vi "open.vi"(11 "Experience ID":string="TestOK") -> (0 "error out":errorcluster, 2 "Indicators_list":T1(array[cluster]), 3 "Controls_list":T1(array[cluster]))   [LabVIEW 2014]
panel:
  out "Control Value:Get All":cluster{"Name":string, "Variant Data":variant}[](array[cluster])
  out "vi reference":refnum<vi>
  in  "OpenFP":bool=TRUE
  # "Open"
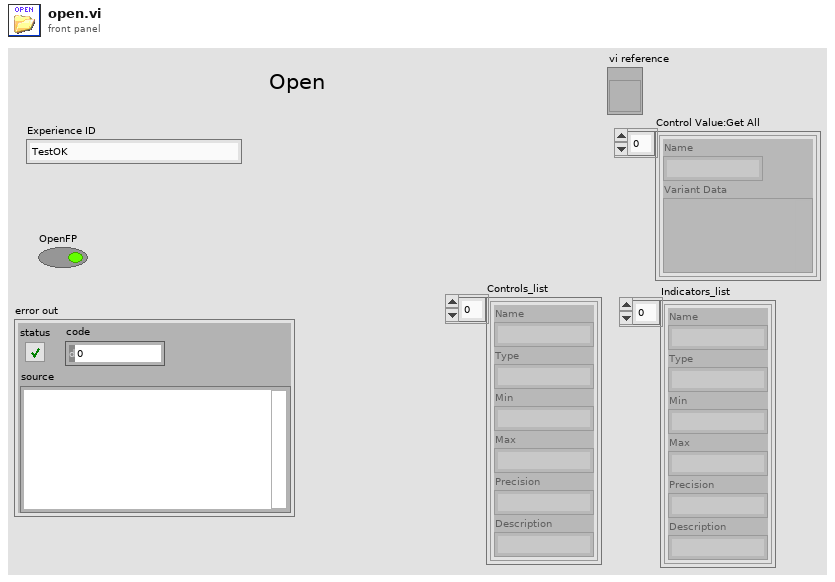
[diagram p1: front panel]
types:
  T1 = cluster{"Name":string, "Type":string, "Min":string, "Max":string, "Precision":string, "Description":string}[]
  T2 = enum32{"Invalid", "Standard", "Closed", "Hidden", "Minimized", "Maximized"}
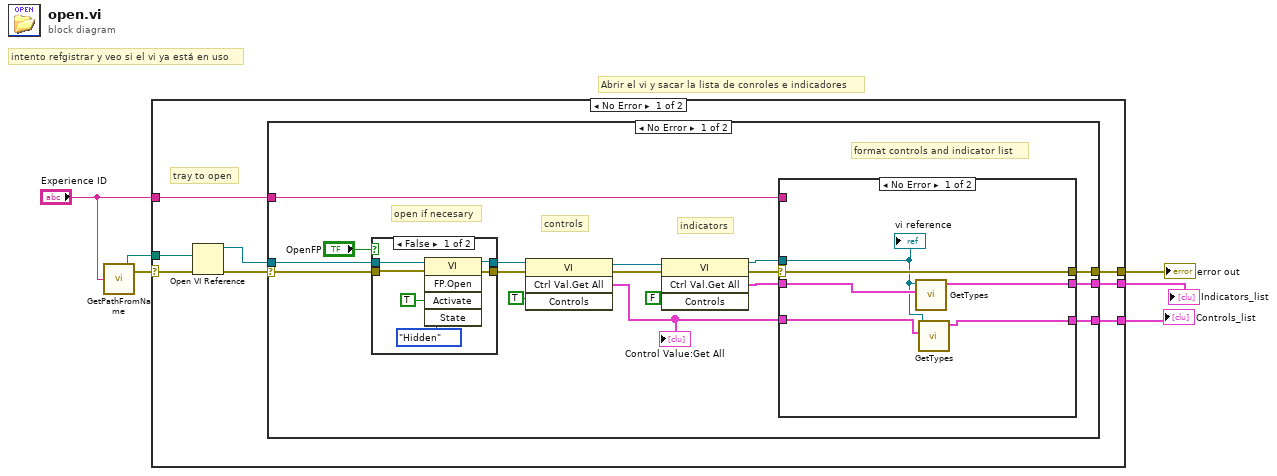
[diagram p0: block diagram]
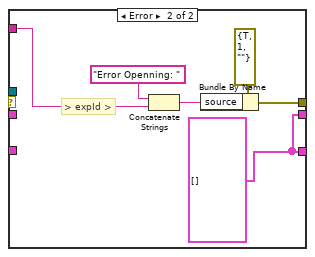
[diagram p2: hidden frame]
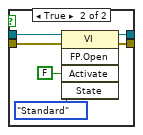
[diagram p3: hidden frame]
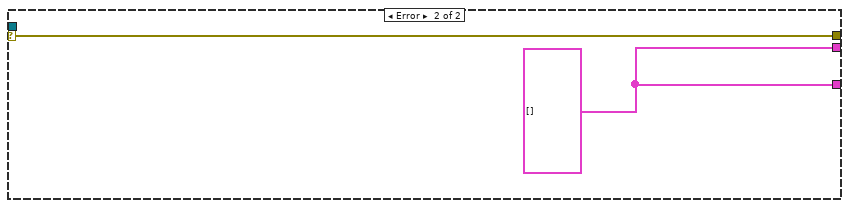
[diagram p4: hidden frame]
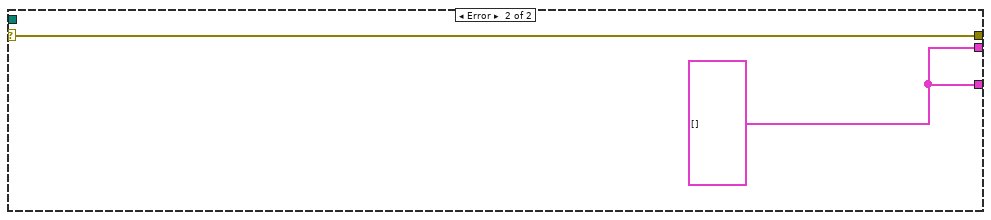
[diagram p5: hidden frame]
diagram:
  # "Abrir el vi y sacar la lista de conroles e indicadores"
  # "intento refgistrar y veo si el vi ya está en uso"
  n1 = call "GetPathFromName.vi"("Experience ID"="Experience ID") -> ("Error out"=w6:errorcluster, "VI_Path"=w5:path)
  n2 = case shown="No Error" w6 {
    selector: w6 -> [w14 w59]
    tunnel: w5 -> [w13 _]
    tunnel: "Experience ID" -> [w10 _]
    tunnel: [w9 w59] -> w3
    tunnel: [w8 w58] -> w1
    tunnel: [w7 w58] -> w2
    frame No Error {
      # "tray to open"
      n3 = Open VI Reference(vi path=w13, error in (no error)=w14) -> (vi reference=w12:refnum<vi>, error out=w11:errorcluster)  [unwired: 1 in, 3 out]
      n4 = case shown="No Error" w11 {
        selector: w11 -> [w27 w57]
        tunnel: w12 -> [w28 _]
        tunnel: w10 -> [w30 _]
        tunnel: [w29 w57] -> w9
        tunnel: [w18 w56] -> w8
        tunnel: [w17 w56] -> w7
        frame No Error {
          # "indicators"
          # "controls"
          # "open if necesary"
          # "format controls and indicator list"
          n5 = case shown="False" "OpenFP" {
            tunnel: w28 -> [w46 w55]
            tunnel: w27 -> [w47 w54]
            tunnel: [w48 w53] -> w22
            tunnel: [w49 w52] -> w23
            frame False {
              n6 = invoke class="VI" method="FP.Open"(reference=w46, error in=w47, "Activate"=TRUE ("Activate?"), "State"=T2."Hidden") -> (reference out=w49:refnum<vi>, error out=w48:errorcluster)  [unwired: 1 in, 3 out]
            }
            frame True {
              n7 = invoke class="VI" method="FP.Open"(reference=w55, error in=w54, "Activate"=FALSE ("Activate?"), "State"=T2."Standard") -> (reference out=w52:refnum<vi>, error out=w53:errorcluster)  [unwired: 1 in, 3 out]
            }
          }
          n8 = invoke class="VI" method="Ctrl Val.Get All"(reference=w23, error in=w22, "Controls"=TRUE) -> (reference out=w15:refnum<vi>, error out=w25:errorcluster, "Get All Control Values Variant"=w19:cluster{"Name":string, "Variant Data":variant}[])  [unwired: 1 in, 1 out]
          "Control Value:Get All" <- w19
          n9 = invoke class="VI" method="Ctrl Val.Get All"(reference=w15, error in=w25, "Controls"=FALSE) -> (reference out=w16:refnum<vi>, error out=w21:errorcluster, "Get All Control Values Variant"=w20:cluster{"Name":string, "Variant Data":variant}[])  [unwired: 1 in, 1 out]
          n10 = case shown="No Error" w21 {
            selector: w21 -> [w37 _]
            tunnel: w30 -> [_ w39]
            tunnel: [w37 w43] -> w29
            tunnel: w19 -> [w34 _]
            tunnel: w20 -> [w36 _]
            tunnel: [w32 w38] -> w18
            tunnel: [w35 w38] -> w17
            tunnel: w16 -> [w33 _]
            frame No Error {
              n11 = call "GetTypes.vi"("vi reference"=w33, "controls or indicators"=w36) -> ("types"=w35:T1)  [unwired: 8 in]
              n12 = call "GetTypes.vi"("vi reference"=w33, "controls or indicators"=w34) -> ("types"=w32:T1)  [unwired: 8 in]
              "vi reference" <- w33
            }
            frame Error {
              w38 = T1 [] ("Control types")
              # "> expId >"
              n13 = Concatenate Strings("Error Openning: " ("string"), w39) -> (w41:string)
              n14 = Bundle By Name(cluster=errorcluster {"status"=TRUE, "code"=1, "source"=""} ("Error"), "source"=w41) -> (w43:errorcluster)
            }
          }
        }
        frame Error {
          w56 = T1 [] ("Control types")
        }
      }
    }
    frame Error {
      w58 = T1 [] ("Control types")
    }
  }
  "error out" <- w3
  "Indicators_list" <- w2
  "Controls_list" <- w1
